vi "Generate Resource Name.vi"(8 "error in (no error)":errorcluster, 11 "SLSC Switch Custom Device Ref in":u64) -> (0 "error out":errorcluster, 2 "Resource Name":string, 3 "SLSC Switch Custom Device Ref out":u64)   [LabVIEW 2017, in "SLSC Switch System Explorer.lvlib"]
uses:
  SLSC Switch System Explorer.lvlib
  <vilib>/NI Veristand/Custom Device Tools/Custom Device Utility Library/Search Direction.ctl
  Scripting/SLSC Scripting Constants.vi
  Scripting/SLSC Switch Scripting.lvlib
  <vilib>/NI Veristand/Custom Device Tools/Custom Device Utility Library/Custom Device Utility Library.lvlib
  <vilib>/NI Veristand/Custom Device API/Custom Device API.lvlib
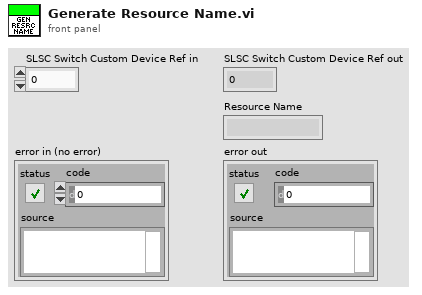
[diagram p1: front panel]
types:
  T1 = typedef "Custom Device Utility Library.lvlib/Search Direction.ctl" = enum16{"Down", "Up"}
  T2 = typedef "Custom Device API.lvlib/Custom Device Item Ref.ctl" = u64
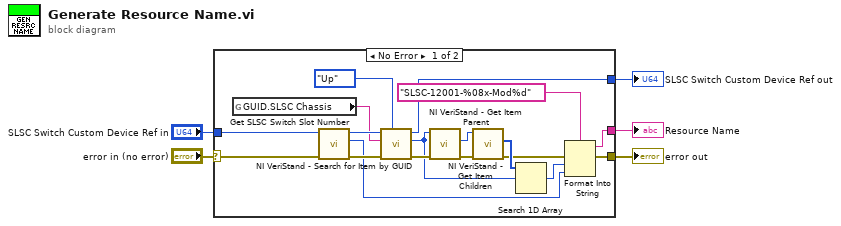
[diagram p0: block diagram]
diagram:
  n1 = case shown="No Error" "error in (no error)" {
    selector: "error in (no error)" -> [w23 w24]
    tunnel: [w10 w24] -> w4
    tunnel: [w6 w25] -> w3
    tunnel: "SLSC Switch Custom Device Ref in" -> [w22 w25]
    tunnel: [w7 _] -> w1
    frame No Error {
      n2 = global read "SLSC Scripting Constants.vi" "GUID.SLSC Chassis"() -> (w14:string)
      n3 = call "Get SLSC Switch Slot Number.vi"("error in (no error)"=w23, "SLSC Switch Custom Device Ref in"=w22) -> ("error out"=w17:errorcluster, "Slot Number"=w8:i32, "SLSC Switch Custom Device Ref out"=w18:T2)  [unwired: 7 in]
      n4 = call <vilib>:"NI VeriStand - Search for Item by GUID.vi"("Direction (Down)"=Search_Direction."Up", "error in"=w17, "Item GUID"=w14, "Section Ref in"=w18) -> ("error out"=w19:errorcluster, "Item Ref"=w13:T2, "Section Ref out"=w6:T2)  [unwired: 4 in, 1 out]
      n5 = call <vilib>:"NI VeriStand - Get Item Parent.vi"("error in (no error)"=w19, "Item Ref in"=w13) -> ("error out"=w16:errorcluster, "Parent Ref"=w21:T2)  [unwired: 6 in, 2 out]
      n6 = call <vilib>:"NI VeriStand - Get Item Children.vi"("error in (no error)"=w16, "Item Ref in"=w21) -> ("error out"=w11:errorcluster, "Child Refs"=w20:T2[])  [unwired: 6 in, 2 out]
      n7 = Search 1D Array(1D array=w20, element=w13) -> (index of element=w9:i32)  [unwired: 1 in]
      n8 = Format Into String(format string="SLSC-12001-%08x-Mod%d", error in=w11, w9, w8) -> (resulting string=w7:string, error out=w10:errorcluster)  [unwired: 1 in]
    }
    frame Error {
    }
  }
  "SLSC Switch Custom Device Ref out" <- w3
  "error out" <- w4
  "Resource Name" <- w1
